vi "Read RI and DFI Mode.vi"(8 "error in (no error)":errorcluster, 11 "VISA resource name":refnum<visa-resource-name>) -> (0 "error out":errorcluster, 1 "DFI Source Response":string, 2 "RI Mode Response":string, 3 "VISA resource name out":refnum<visa-resource-name>)   [LabVIEW 2021, in "Keithley 2200 Series.lvlib"]
doc: "Returns the output state of the power supply or \nindicate the reason for internal failure."
uses:
  <instrlib>/Keithley 2200 Series/Keithley 2200 Series.lvlib
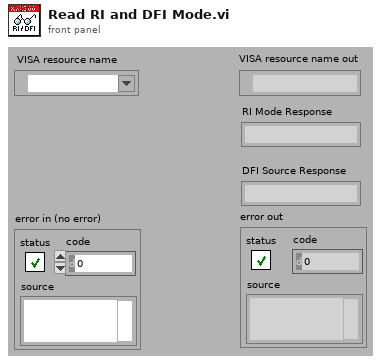
[diagram p1: front panel]
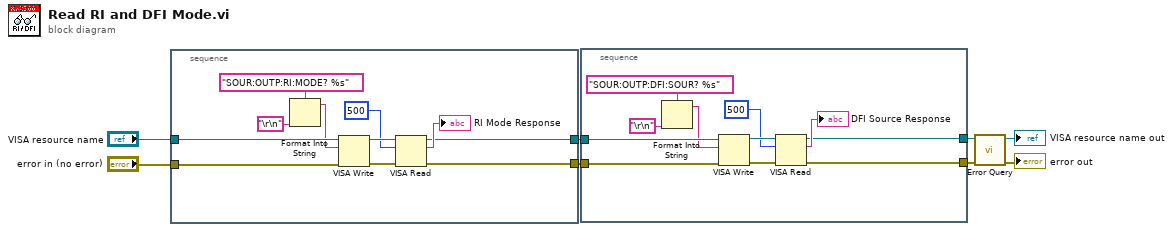
[diagram p0: block diagram]
diagram:
  n1 = stacked-sequence {
    tunnel: "VISA resource name" -> [w19]
    tunnel: "error in (no error)" -> [w18]
    tunnel: [w13] -> w4
    tunnel: [w12] -> w3
    frame #0 {
      n2 = Format Into String(format string="SOUR:OUTP:RI:MODE? %s", "\r\n") -> (resulting string=w9:string)  [unwired: 2 in, 1 out]
      n3 = VISA Write(VISA resource name=w19, write buffer=w9, error in (no error)=w18) -> (VISA resource name out=w17:refnum<visa-resource-name>, error out=w16:errorcluster)  [unwired: 1 out]
      n4 = VISA Read(VISA resource name=w17, byte count=u32 500, error in (no error)=w16) -> (VISA resource name out=w13:refnum<visa-resource-name>, read buffer=→"RI Mode Response":string, error out=w12:errorcluster)  [unwired: 1 out]
    }
  }
  n5 = stacked-sequence {
    tunnel: w4 -> [w30]
    tunnel: w3 -> [w29]
    tunnel: [w24] -> w2
    tunnel: [w23] -> w1
    frame #0 {
      n6 = Format Into String(format string="SOUR:OUTP:DFI:SOUR? %s", "\r\n") -> (resulting string=w20:string)  [unwired: 2 in, 1 out]
      n7 = VISA Write(VISA resource name=w30, write buffer=w20, error in (no error)=w29) -> (VISA resource name out=w28:refnum<visa-resource-name>, error out=w27:errorcluster)  [unwired: 1 out]
      n8 = VISA Read(VISA resource name=w28, byte count=u32 500, error in (no error)=w27) -> (VISA resource name out=w24:refnum<visa-resource-name>, read buffer=→"DFI Source Response":string, error out=w23:errorcluster)  [unwired: 1 out]
    }
  }
  n9 = call <instrlib>:"Error Query.vi"("error in (no error)"=w1, "VISA resource name"=w2) -> ("error out"=→"error out":errorcluster, "VISA resource name out"=→"VISA resource name out":refnum<visa-resource-name>)  [unwired: 8 out]
